vi "timekeeper gain controller.vi"(8 "offset":fxp<+/-,24,24>) -> (3 "adjustment rate (ns/s)":fxp<+/-,21,21>)   [LabVIEW 2011, in "EPS_Timekeeper.lvlib"]
uses:
  <vilib>/addons/Electrical Power/Example Support/PMU/Time Keeper/EPS_Timekeeper.lvlib
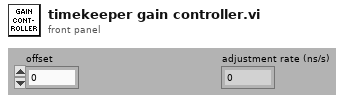
[diagram p1: front panel]
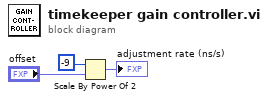
[diagram p0: block diagram]
diagram:
  n1 = Scale By Power Of 2(n=-9 ("denominator"), x="offset") -> (x*2^n=→"adjustment rate (ns/s)":fxp<+/-,24,24>)
